vi "2P_AdapUprite_Linlin.vi"() -> ()   [LabVIEW 2015] (continued)
                        n4091 = control-ref of="Digital Lines Plot"() -> (w894:refnum<vi>)
                        n4092 = local write "Digital Used Lines"(w892) -> ()
                        n4093 = local write "Digital Used Names"(w893) -> ()
                        n4094 = call "prepAOWaveplot.vi"("WaveformGraph in"=w896, "Analog Used Names"=w895) -> ()  [unwired: 1 in]
                        n4095 = call "prepDOWaveplot.vi"("DigitalGraph in"=w894, "used DO names"=w893) -> ()  [unwired: 1 in]
                      }
                    }
                  }
                  frame #4 {
                    n4096 = local read "remDO"() -> (w899:bool)
                    n4097 = case shown="True" w899 {
                      tunnel: w898 -> [_ w900]
                      frame False {
                      }
                      frame True {
                        n4098 = call "waveformparamsv2.vi"("command"="rem DO", "index"=w900) -> ()  [unwired: 3 in, 3 out]
                      }
                    }
                  }
                  frame #5 {
                    n4099 = local read "Meastab"() -> (w905:enum32{"X-Y Image", "Linescan", "Timetrace"})
                    n4100 = property on="refwf" class="Ring (strict)"() -> ("RingText.Text"=w912:string)  [unwired: 2 in, 2 out]
                    n4101 = call "waveformsDObuffer.vi"("command"="get") -> ("DO wf out"=w911:digitalwaveform[])  [unwired: 1 in]
                    n4102 = case shown="\"Timetrace\"" w905 {
                      tunnel: [w921 w922] -> w904
                      frame "X-Y Image", Default {
                        n4103 = local read "Sampling rate"() -> (w921:dbl)
                      }
                      frame "Timetrace" {
                        n4104 = local read "srateAODOtt"() -> (w922:dbl)
                      }
                    }
                    n4105 = call "waveformsAObuffer.vi"("command"="get") -> ("AO wf out"=w920:waveform(dbl)[])  [unwired: 1 in]
                    n4106 = Delete From Array(array=w911, length=1, index=w909) -> (array with subset deleted=w908:digitalwaveform[])  [unwired: 1 out]
                    n4107 = call "correctwaveformsizetemp.vi"("new sampling frequency (Hz)"=w904, "start"=FALSE, "reference waveforms to"=w912, "Analog waveforms in"=w920, "stop"=FALSE, "Digital waveforms in"=w908) -> ("analog wf out"=w915:waveform(dbl)[], "Digital wf out"=w913:digitalwaveform[], "measpoints"=w906:i32)
                    n4108 = local read "wavdet"() -> (w907:bool)
                    n4109 = call "waveformsAObuffer.vi"("AO wf in"=w915, "command"="set") -> ()  [unwired: 1 out]
                    n4110 = call "waveformsDObuffer.vi"("DO wf in"=w913, "command"="set") -> ()  [unwired: 1 out]
                    n4111 = local write "Analog Lines Plot"(w915) -> ()
                    n4112 = local write "Digital Lines Plot"(w913) -> ()
                    n4113 = call "GetNumCamFramesv2.vi"("Digital Waveform Graph"=w913) -> ("Numeric"=w914:i32)  [unwired: 10 in]
                    n4114 = case shown="True" w907 {
                      tunnel: w906 -> [_ w923]
                      frame False {
                      }
                      frame True {
                        n4115 = local write "# of frames"(w923) -> ()
                      }
                    }
                    n4116 = local write "Total Camera Frames"(w914) -> ()
                  }
                  frame #6 {
                    w924 = FALSE ("addAO")
                    n4117 = local read "finite samples"() -> (w925:bool)
                    n4118 = local read "continuous"() -> (w926:bool)
                    n4119 = local read "wavdet"() -> (w927:bool)
                    n4120 = local write "remDO"(w924) -> ()
                    n4121 = call "2pparameters.vi"("command"="get") -> ("params out"=w930:T12)  [unwired: 1 in]
                    n4122 = Bundle By Name(cluster=w930, "finite"=w925, "cont"=w926, "wavdet"=w927) -> (w928:T12)
                    n4123 = property on="Rem DO wave" class="Bool (strict)"("Val(Sgnl)"=w924) -> ()  [unwired: 2 in, 2 out]
                    n4124 = call "2pparameters.vi"("Params in"=w928, "command"="set") -> ()  [unwired: 1 out]
                  }
                }
              }
            }
          }
          event "load changed DO wave": Value Change {
            n4125 = event-data() -> ("NewVal"=w932:bool)  [unwired: 1 in, 5 out]
            n4126 = case shown="True" w932 {
              frame False {
              }
              frame True {
                n4127 = stacked-sequence {
                  seq-local: [_ _ w1040 _ _] -> [_ _ _ w1057 _]
                  seq-local: [_ _ w1039 _ _] -> [_ _ _ w1056 _]
                  frame #0 {
                    n4128 = local read "Measurement"() -> (w934:T4)
                    n4129 = local write "changeDO"(TRUE ("addAO")) -> ()
                    n4130 = case shown="\"X-Y-t movie\", Default" w934 {
                      frame "X-Y-t movie", Default {
                        n4131 = local read "avpp"() -> (w955:i32)
                        n4132 = local read "Angle ref"() -> (w954:dbl)
                        n4133 = local read "ROI Type"() -> (w953:u16)
                        n4134 = local read "xpixels ref"() -> (w950:i32)
                        n4135 = local read "Vx-min ref"() -> (w949:dbl)
                        n4136 = local read "Vx-max ref"() -> (w948:dbl)
                        n4137 = local read "ypixels ref"() -> (w946:i32)
                        n4138 = local read "Vy-min ref"() -> (w947:dbl)
                        n4139 = local read "Vy-max ref"() -> (w943:dbl)
                        n4140 = local read "Sampling rate"() -> (w937:dbl)
                        n4141 = local read "finite samples"() -> (w938:bool)
                        n4142 = local read "continuous"() -> (w941:bool)
                        n4143 = local read "wavdet"() -> (w942:bool)
                        n4144 = local read "# of frames"() -> (w940:i32)
                        n4145 = local read "maxbufferAI"() -> (w939:i32)
                        n4146 = local read "Override AI buffer"() -> (w935:bool)
                        n4147 = call "2pparameters.vi"("command"="get") -> ("params out"=w952:T12)  [unwired: 1 in]
                        n4148 = Bundle By Name(cluster=w952, "type"="X-Y-t movie", "avpp"=w955, "Angle Img"=w954, "Xpixels Img"=w950, "Vx-min Img"=w949, "VX-max Img"=w948, "Ypixels Img"=w946, "Vy-min Img"=w947, "Vy-max Img"=w943, "srate"=w937, "srate Img"=w937, "finite"=w938, "cont"=w941, "wavdet"=w942, "measpoints"=w940, "maxbufferAI"=w939, "Drawing Mode"=w953, "Vz-reset"=0.0, "AIoverride"=w935) -> (w944:T12)
                        n4149 = call "2pparameters.vi"("Params in"=w944, "command"="set") -> ()  [unwired: 1 out]
                      }
                      frame "X-Y-Z stack" {
                        n4150 = call "2pparameters.vi"("command"="get") -> ("params out"=w959:T12)  [unwired: 1 in]
                        n4151 = Bundle By Name(cluster=w959, "type"="X-Y-Z stack") -> (w957:T12)
                        n4152 = call "2pparameters.vi"("Params in"=w957, "command"="set") -> ()  [unwired: 1 out]
                      }
                      frame "Lifetime (scan)" {
                        n4153 = call "2pparameters.vi"("command"="get") -> ("params out"=w964:T12)  [unwired: 1 in]
                        n4154 = Bundle By Name(cluster=w964, "type"="Lifetime (scan)") -> (w962:T12)
                        n4155 = call "2pparameters.vi"("Params in"=w962, "command"="set") -> ()  [unwired: 1 out]
                      }
                      frame "Lifetime (contour)" {
                        n4156 = local read "Vy-min draw"() -> (w974:dbl)
                        n4157 = local read "Vy-max draw"() -> (w973:dbl)
                        n4158 = local read "Vx-min draw"() -> (w976:dbl)
                        n4159 = local read "Vx-max draw"() -> (w975:dbl)
                        n4160 = local read "xpixels ref"() -> (w972:i32)
                        n4161 = local read "ypixels ref"() -> (w971:i32)
                        n4162 = local read "ROI Type"() -> (w970:u16)
                        n4163 = local read "srateAODOtt"() -> (w981:dbl)
                        n4164 = local read "# of frames"() -> (w986:i32)
                        n4165 = local read "refreshtime"() -> (w978:dbl)
                        n4166 = local read "Pel"() -> (w969:dbl)
                        n4167 = local read "bin"() -> (w984:dbl)
                        n4168 = local read "Override AI buffer"() -> (w967:bool)
                        n4169 = local read "finite samples"() -> (w993:bool)
                        n4170 = local read "srateAODOtt"() -> (w980:dbl)
                        n4171 = local read "srateAODOtt"() -> (w987:dbl)
                        n4172 = local read "continuous"() -> (w992:bool)
                        n4173 = local read "Angle ref"() -> (w977:dbl)
                        n4174 = local read "wavdet"() -> (w994:bool)
                        n4175 = local read "Vx-ref"() -> (w989:dbl)
                        n4176 = local read "Vy-ref"() -> (w991:dbl)
                        n4177 = local read "avpp"() -> (w990:i32)
                        n4178 = call "tt_timeandsamples.vi"("bin"=w984, "refreshtime"=w978, "srateAODOtt"=w981, "tot#ofsamples"=w986) -> ("refreshrate"=w982:dbl, "refreshbuffer"=w983:i32, "timetracecycles"=w988:i32)  [unwired: 5 in]
                        n4179 = local read "bin"() -> (w985:dbl)
                        n4180 = call "2pparameters.vi"("command"="get") -> ("params out"=w997:T12)  [unwired: 1 in]
                        n4181 = Bundle By Name(cluster=w997, "Drawing Mode"=w970, "measpoints"=w986, "tt_cycles"=w988, "refreshbuffer"=w983, "refreshrate"=w982, "Vx-ref"=w989, "Vy-ref"=w991, "srate"=w980, "finite"=w993, "cont"=w992, "wavdet"=w994, "avpp"=w990, "srateAODO"=w987, "bufferAI"=w983, "bin"=w985, "Angle Img"=w977, "Vxminref"=w976, "Vxmaxref"=w975, "Vyminref"=w974, "Vymaxref"=w973, "Xpixels Img"=w972, "Ypixels Img"=w971, "Pel"=w969, "Vz-reset"=0.0, "AIoverride"=w967, "type"="Lifetime (contour)") -> (w995:T12)
                        n4182 = Reciprocal(x=w982) -> (1/x=w979:dbl)
                        n4183 = local write "refreshtime"(w979) -> ()
                        n4184 = call "2pparameters.vi"("Params in"=w995, "command"="set") -> ()  [unwired: 1 out]
                      }
                      frame "X-Y-Z-t movie" {
                      }
                      frame "linescan" {
                      }
                      frame "Timetrace" {
                        n4185 = local read "Vy-min draw"() -> (w1007:dbl)
                        n4186 = local read "Vy-max draw"() -> (w1006:dbl)
                        n4187 = local read "Vx-min draw"() -> (w1009:dbl)
                        n4188 = local read "Vx-max draw"() -> (w1008:dbl)
                        n4189 = local read "xpixels ref"() -> (w1005:i32)
                        n4190 = local read "ypixels ref"() -> (w1004:i32)
                        n4191 = local read "ROI Type"() -> (w1003:u16)
                        n4192 = local read "srateAODOtt"() -> (w1014:dbl)
                        n4193 = local read "# of frames"() -> (w1019:i32)
                        n4194 = local read "refreshtime"() -> (w1011:dbl)
                        n4195 = local read "Pel"() -> (w1002:dbl)
                        n4196 = local read "bin"() -> (w1017:dbl)
                        n4197 = local read "Override AI buffer"() -> (w1000:bool)
                        n4198 = local read "finite samples"() -> (w1026:bool)
                        n4199 = local read "srateAODOtt"() -> (w1013:dbl)
                        n4200 = local read "srateAODOtt"() -> (w1020:dbl)
                        n4201 = local read "continuous"() -> (w1025:bool)
                        n4202 = local read "Angle ref"() -> (w1010:dbl)
                        n4203 = local read "wavdet"() -> (w1027:bool)
                        n4204 = local read "Vx-ref"() -> (w1022:dbl)
                        n4205 = local read "Vy-ref"() -> (w1024:dbl)
                        n4206 = local read "avpp"() -> (w1023:i32)
                        n4207 = call "tt_timeandsamples.vi"("bin"=w1017, "refreshtime"=w1011, "srateAODOtt"=w1014, "tot#ofsamples"=w1019) -> ("refreshrate"=w1015:dbl, "refreshbuffer"=w1016:i32, "timetracecycles"=w1021:i32)  [unwired: 5 in]
                        n4208 = local read "bin"() -> (w1018:dbl)
                        n4209 = call "2pparameters.vi"("command"="get") -> ("params out"=w1030:T12)  [unwired: 1 in]
                        n4210 = Bundle By Name(cluster=w1030, "Drawing Mode"=w1003, "measpoints"=w1019, "tt_cycles"=w1021, "refreshbuffer"=w1016, "refreshrate"=w1015, "Vx-ref"=w1022, "Vy-ref"=w1024, "srate"=w1013, "finite"=w1026, "cont"=w1025, "wavdet"=w1027, "avpp"=w1023, "srateAODO"=w1020, "bufferAI"=w1016, "bin"=w1018, "Angle Img"=w1010, "Vxminref"=w1009, "Vxmaxref"=w1008, "Vyminref"=w1007, "Vymaxref"=w1006, "Xpixels Img"=w1005, "Ypixels Img"=w1004, "Pel"=w1002, "Vz-reset"=0.0, "AIoverride"=w1000, "type"="Timetrace") -> (w1028:T12)
                        n4211 = Reciprocal(x=w1015) -> (1/x=w1012:dbl)
                        n4212 = local write "refreshtime"(w1012) -> ()
                        n4213 = call "2pparameters.vi"("Params in"=w1028, "command"="set") -> ()  [unwired: 1 out]
                      }
                      frame "Lifetime (point)" {
                      }
                    }
                  }
                  frame #1 {
                    w1033 = FALSE ("wavdet")
                    n4214 = call "2pparameters.vi"("command"="get") -> ("params out"=w1037:T12)  [unwired: 1 in]
                    n4215 = Bundle By Name(cluster=w1037, "finite"=w1033, "cont"=w1033, "wavdet"=TRUE) -> (w1034:T12)
                    n4216 = call "2pparameters.vi"("Params in"=w1034, "command"="set") -> ()  [unwired: 1 out]
                  }
                  frame #2 {
                    n4217 = local read "DO channels"() -> (w1042:u16)
                    n4218 = call "2pparameters.vi"("command"="get") -> ("params out"=w1044:T12)  [unwired: 1 in]
                    n4219 = Unbundle By Name(w1044) -> ("aDO"=w1043:u32[])
                    n4220 = Search 1D Array(1D array=w1043, element=w1042) -> (index of element=w1040:i32)  [unwired: 1 in]
                    n4221 = Greater?(x=w1040, y=-1) -> (0:w1039:bool)
                    n4222 = case shown="True" w1039 {
                      tunnel: w1040 -> [_ w1053]
                      frame False {
                      }
                      frame True {
                        n4223 = local read "Meastab"() -> (w1047:enum32{"X-Y Image", "Linescan", "Timetrace"})
                        n4224 = local read "Digital padding value"() -> (w1048:dbl)
                        n4225 = local read "Digital time offset (s)"() -> (w1049:dbl)
                        n4226 = case shown="\"Timetrace\"" w1047 {
                          tunnel: [w1054 w1055] -> w1046
                          frame "X-Y Image", Default {
                            n4227 = local read "Sampling rate"() -> (w1054:dbl)
                          }
                          frame "Timetrace" {
                            n4228 = local read "srateAODOtt"() -> (w1055:dbl)
                          }
                        }
                        n4229 = local read "Digital Freq (Hz)"() -> (w1051:dbl)
                        n4230 = local read "Digital phase (s)"() -> (w1050:dbl)
                        n4231 = local read "Digital DC (%)"() -> (w1052:dbl)
                        n4232 = call "replace DO wf param.vi"("Digital Freq (Hz)"=w1051, "Digital DC (%)"=w1052, "Digital phase"=w1050, "Sampling frequency (Hz)"=w1046, "Digital time offset (s)"=w1049, "index of DO wave"=w1053, "padding value"=w1048) -> ()  [unwired: 4 in]
                      }
                    }
                  }
                  frame #3 {
                    n4233 = case shown="True" w1056 {
                      tunnel: w1057 -> [_ w1064]
                      frame False {
                      }
                      frame True {
                        n4234 = local read "Meastab"() -> (w1061:enum32{"X-Y Image", "Linescan", "Timetrace"})
                        n4235 = call "waveformparamsv2.vi"("command"="get") -> ("Params out"=w1080:T17)  [unwired: 4 in, 2 out]
                        n4236 = Unbundle By Name(w1080) -> ("DO parameters"=w1079:T20)
                        n4237 = property on="refwf" class="Ring (strict)"() -> ("RingText.Text"=w1086:string)  [unwired: 2 in, 2 out]
                        n4238 = case shown="\"Timetrace\"" w1061 {
                          tunnel: [w1087 w1088] -> w1060
                          frame "X-Y Image", Default {
                            n4239 = local read "Sampling rate"() -> (w1087:dbl)
                          }
                          frame "Timetrace" {
                            n4240 = local read "srateAODOtt"() -> (w1088:dbl)
                          }
                        }
                        n4241 = call "waveformsAObuffer.vi"("command"="get") -> ("AO wf out"=w1084:waveform(dbl)[])  [unwired: 1 in]
                        n4242 = call "waveformsDObuffer.vi"("command"="get") -> ("DO wf out"=w1082:digitalwaveform[])  [unwired: 1 in]
                        n4243 = call "referfencesize.vi"("Digital waveforms in"=w1082, "Analog waveforms in"=w1084, "reference waveforms to"=w1086) -> ("number of samples"=w1077:i32)  [unwired: 2 in]
                        n4244 = Index Array(array=w1079, index=w1064) -> (element=w1078:T21)
                        n4245 = call "waveformsDObuffer.vi"("command"="get") -> ("DO wf out"=w1074:digitalwaveform[])  [unwired: 1 in]
                        n4246 = call "simple digital from wf params.vi"("waveform params"=w1078, "number of samples"=w1077) -> ("digital waveform"=w1076:digitalwaveform)
                        n4247 = property on="refwf" class="Ring (strict)"() -> ("RingText.Text"=w1066:string)  [unwired: 2 in, 2 out]
                        n4248 = Replace Array Subset(array=w1074, new element=w1076, index=w1064) -> (w1065:digitalwaveform[])
                        n4249 = call "waveformsAObuffer.vi"("command"="get") -> ("AO wf out"=w1073:waveform(dbl)[])  [unwired: 1 in]
                        n4250 = local read "wavdet"() -> (w1063:bool)
                        n4251 = call "correctwaveformsizetemp.vi"("new sampling frequency (Hz)"=w1060, "start"=FALSE, "reference waveforms to"=w1066, "Analog waveforms in"=w1073, "stop"=FALSE, "Digital waveforms in"=w1065) -> ("analog wf out"=w1069:waveform(dbl)[], "Digital wf out"=w1067:digitalwaveform[], "measpoints"=w1062:i32)
                        n4252 = local write "Analog Lines Plot"(w1069) -> ()
                        n4253 = call "GetNumCamFramesv2.vi"("Digital Waveform Graph"=w1067) -> ("Numeric"=w1068:i32)  [unwired: 10 in]
                        n4254 = local write "Digital Lines Plot"(w1067) -> ()
                        n4255 = case shown="True" w1063 {
                          tunnel: w1062 -> [_ w1089]
                          frame False {
                          }
                          frame True {
                            n4256 = local write "# of frames"(w1089) -> ()
                          }
                        }
                        n4257 = call "waveformsAObuffer.vi"("AO wf in"=w1069, "command"="set") -> ()  [unwired: 1 out]
                        n4258 = call "waveformsDObuffer.vi"("DO wf in"=w1067, "command"="set") -> ()  [unwired: 1 out]
                        n4259 = local write "Total Camera Frames"(w1068) -> ()
                      }
                    }
                  }
                  frame #4 {
                    w1091 = FALSE ("addAO")
                    n4260 = local read "finite samples"() -> (w1092:bool)
                    n4261 = local read "continuous"() -> (w1093:bool)
                    n4262 = local read "wavdet"() -> (w1094:bool)
                    n4263 = local write "changeDO"(w1091) -> ()
                    n4264 = property on="load changed DO wave" class="Bool (strict)"("Val(Sgnl)"=w1091) -> ()  [unwired: 2 in, 2 out]
                    n4265 = call "2pparameters.vi"("command"="get") -> ("params out"=w1097:T12)  [unwired: 1 in]
                    n4266 = Bundle By Name(cluster=w1097, "finite"=w1092, "cont"=w1093, "wavdet"=w1094) -> (w1095:T12)
                    n4267 = local write "not loadedDO"(FALSE ("not loadedDO")) -> ()
                    n4268 = call "2pparameters.vi"("Params in"=w1095, "command"="set") -> ()  [unwired: 1 out]
                  }
                }
              }
            }
          }
          event "refwf": Value Change {
            n4269 = event-data() -> ()  [unwired: 1 in, 6 out]
            n4270 = stacked-sequence {
              frame #0 {
                n4271 = local read "Measurement"() -> (w1099:T4)
                n4272 = case shown="\"Timetrace\"" w1099 {
                  frame "X-Y-t movie", Default {
                    n4273 = local read "avpp"() -> (w1120:i32)
                    n4274 = local read "Angle ref"() -> (w1119:dbl)
                    n4275 = local read "ROI Type"() -> (w1118:u16)
                    n4276 = local read "xpixels ref"() -> (w1115:i32)
                    n4277 = local read "Vx-min ref"() -> (w1114:dbl)
                    n4278 = local read "Vx-max ref"() -> (w1113:dbl)
                    n4279 = local read "ypixels ref"() -> (w1111:i32)
                    n4280 = local read "Vy-min ref"() -> (w1112:dbl)
                    n4281 = local read "Vy-max ref"() -> (w1108:dbl)
                    n4282 = local read "Sampling rate"() -> (w1102:dbl)
                    n4283 = local read "finite samples"() -> (w1103:bool)
                    n4284 = local read "continuous"() -> (w1106:bool)
                    n4285 = local read "wavdet"() -> (w1107:bool)
                    n4286 = local read "# of frames"() -> (w1105:i32)
                    n4287 = local read "maxbufferAI"() -> (w1104:i32)
                    n4288 = local read "Override AI buffer"() -> (w1100:bool)
                    n4289 = call "2pparameters.vi"("command"="get") -> ("params out"=w1117:T12)  [unwired: 1 in]
                    n4290 = Bundle By Name(cluster=w1117, "type"="X-Y-t movie", "avpp"=w1120, "Angle Img"=w1119, "Xpixels Img"=w1115, "Vx-min Img"=w1114, "VX-max Img"=w1113, "Ypixels Img"=w1111, "Vy-min Img"=w1112, "Vy-max Img"=w1108, "srate"=w1102, "srate Img"=w1102, "finite"=w1103, "cont"=w1106, "wavdet"=w1107, "measpoints"=w1105, "maxbufferAI"=w1104, "Drawing Mode"=w1118, "Vz-reset"=0.0, "AIoverride"=w1100) -> (w1109:T12)
                    n4291 = call "2pparameters.vi"("Params in"=w1109, "command"="set") -> ()  [unwired: 1 out]
                  }
                  frame "X-Y-Z stack" {
                    n4292 = call "2pparameters.vi"("command"="get") -> ("params out"=w1124:T12)  [unwired: 1 in]
                    n4293 = Bundle By Name(cluster=w1124, "type"="X-Y-Z stack") -> (w1122:T12)
                    n4294 = call "2pparameters.vi"("Params in"=w1122, "command"="set") -> ()  [unwired: 1 out]
                  }
                  frame "Lifetime (scan)" {
                    n4295 = call "2pparameters.vi"("command"="get") -> ("params out"=w1129:T12)  [unwired: 1 in]
                    n4296 = Bundle By Name(cluster=w1129, "type"="Lifetime (scan)") -> (w1127:T12)
                    n4297 = call "2pparameters.vi"("Params in"=w1127, "command"="set") -> ()  [unwired: 1 out]
                  }
                  frame "Lifetime (contour)" {
                    n4298 = local read "Vy-min draw"() -> (w1139:dbl)
                    n4299 = local read "Vy-max draw"() -> (w1138:dbl)
                    n4300 = local read "Vx-min draw"() -> (w1141:dbl)
                    n4301 = local read "Vx-max draw"() -> (w1140:dbl)
                    n4302 = local read "xpixels ref"() -> (w1137:i32)
                    n4303 = local read "ypixels ref"() -> (w1136:i32)
                    n4304 = local read "ROI Type"() -> (w1135:u16)
                    n4305 = local read "srateAODOtt"() -> (w1146:dbl)
                    n4306 = local read "# of frames"() -> (w1151:i32)
                    n4307 = local read "refreshtime"() -> (w1143:dbl)
                    n4308 = local read "Pel"() -> (w1134:dbl)
                    n4309 = local read "bin"() -> (w1149:dbl)
                    n4310 = local read "Override AI buffer"() -> (w1132:bool)
                    n4311 = local read "finite samples"() -> (w1158:bool)
                    n4312 = local read "srateAODOtt"() -> (w1145:dbl)
                    n4313 = local read "srateAODOtt"() -> (w1152:dbl)
                    n4314 = local read "continuous"() -> (w1157:bool)
                    n4315 = local read "Angle ref"() -> (w1142:dbl)
                    n4316 = local read "wavdet"() -> (w1159:bool)
                    n4317 = local read "Vx-ref"() -> (w1154:dbl)
                    n4318 = local read "Vy-ref"() -> (w1156:dbl)
                    n4319 = local read "avpp"() -> (w1155:i32)
                    n4320 = call "tt_timeandsamples.vi"("bin"=w1149, "refreshtime"=w1143, "srateAODOtt"=w1146, "tot#ofsamples"=w1151) -> ("refreshrate"=w1147:dbl, "refreshbuffer"=w1148:i32, "timetracecycles"=w1153:i32)  [unwired: 5 in]
                    n4321 = local read "bin"() -> (w1150:dbl)
                    n4322 = call "2pparameters.vi"("command"="get") -> ("params out"=w1162:T12)  [unwired: 1 in]
                    n4323 = Bundle By Name(cluster=w1162, "Drawing Mode"=w1135, "measpoints"=w1151, "tt_cycles"=w1153, "refreshbuffer"=w1148, "refreshrate"=w1147, "Vx-ref"=w1154, "Vy-ref"=w1156, "srate"=w1145, "finite"=w1158, "cont"=w1157, "wavdet"=w1159, "avpp"=w1155, "srateAODO"=w1152, "bufferAI"=w1148, "bin"=w1150, "Angle Img"=w1142, "Vxminref"=w1141, "Vxmaxref"=w1140, "Vyminref"=w1139, "Vymaxref"=w1138, "Xpixels Img"=w1137, "Ypixels Img"=w1136, "Pel"=w1134, "Vz-reset"=0.0, "AIoverride"=w1132, "type"="Lifetime (contour)") -> (w1160:T12)
                    n4324 = Reciprocal(x=w1147) -> (1/x=w1144:dbl)
                    n4325 = local write "refreshtime"(w1144) -> ()
                    n4326 = call "2pparameters.vi"("Params in"=w1160, "command"="set") -> ()  [unwired: 1 out]
                  }
                  frame "X-Y-Z-t movie" {
                  }
                  frame "linescan" {
                  }
                  frame "Timetrace" {
                    n4327 = local read "Vy-min draw"() -> (w1172:dbl)
                    n4328 = local read "Vy-max draw"() -> (w1171:dbl)
                    n4329 = local read "Vx-min draw"() -> (w1174:dbl)
                    n4330 = local read "Vx-max draw"() -> (w1173:dbl)
                    n4331 = local read "xpixels ref"() -> (w1170:i32)
                    n4332 = local read "ypixels ref"() -> (w1169:i32)
                    n4333 = local read "ROI Type"() -> (w1168:u16)
                    n4334 = local read "srateAODOtt"() -> (w1179:dbl)
                    n4335 = local read "# of frames"() -> (w1184:i32)
                    n4336 = local read "refreshtime"() -> (w1176:dbl)
                    n4337 = local read "Pel"() -> (w1167:dbl)
                    n4338 = local read "bin"() -> (w1182:dbl)
                    n4339 = local read "Override AI buffer"() -> (w1165:bool)
                    n4340 = local read "finite samples"() -> (w1191:bool)
                    n4341 = local read "srateAODOtt"() -> (w1178:dbl)
                    n4342 = local read "srateAODOtt"() -> (w1185:dbl)
                    n4343 = local read "continuous"() -> (w1190:bool)
                    n4344 = local read "Angle ref"() -> (w1175:dbl)
                    n4345 = local read "wavdet"() -> (w1192:bool)
                    n4346 = local read "Vx-ref"() -> (w1187:dbl)
                    n4347 = local read "Vy-ref"() -> (w1189:dbl)
                    n4348 = local read "avpp"() -> (w1188:i32)
                    n4349 = call "tt_timeandsamples.vi"("bin"=w1182, "refreshtime"=w1176, "srateAODOtt"=w1179, "tot#ofsamples"=w1184) -> ("refreshrate"=w1180:dbl, "refreshbuffer"=w1181:i32, "timetracecycles"=w1186:i32)  [unwired: 5 in]
                    n4350 = local read "bin"() -> (w1183:dbl)
                    n4351 = call "2pparameters.vi"("command"="get") -> ("params out"=w1195:T12)  [unwired: 1 in]
                    n4352 = Bundle By Name(cluster=w1195, "Drawing Mode"=w1168, "measpoints"=w1184, "tt_cycles"=w1186, "refreshbuffer"=w1181, "refreshrate"=w1180, "Vx-ref"=w1187, "Vy-ref"=w1189, "srate"=w1178, "finite"=w1191, "cont"=w1190, "wavdet"=w1192, "avpp"=w1188, "srateAODO"=w1185, "bufferAI"=w1181, "bin"=w1183, "Angle Img"=w1175, "Vxminref"=w1174, "Vxmaxref"=w1173, "Vyminref"=w1172, "Vymaxref"=w1171, "Xpixels Img"=w1170, "Ypixels Img"=w1169, "Pel"=w1167, "Vz-reset"=0.0, "AIoverride"=w1165, "type"="Timetrace") -> (w1193:T12)
                    n4353 = Reciprocal(x=w1180) -> (1/x=w1177:dbl)
                    n4354 = local write "refreshtime"(w1177) -> ()
                    n4355 = call "2pparameters.vi"("Params in"=w1193, "command"="set") -> ()  [unwired: 1 out]
                  }
                  frame "Lifetime (point)" {
                  }
                }
              }
              frame #1 {
                w1198 = FALSE ("wavdet")
                n4356 = call "2pparameters.vi"("command"="get") -> ("params out"=w1202:T12)  [unwired: 1 in]
                n4357 = Bundle By Name(cluster=w1202, "finite"=w1198, "cont"=w1198, "wavdet"=TRUE) -> (w1199:T12)
                n4358 = call "2pparameters.vi"("Params in"=w1199, "command"="set") -> ()  [unwired: 1 out]
              }
              frame #2 {
                n4359 = local read "Meastab"() -> (w1207:enum32{"X-Y Image", "Linescan", "Timetrace"})
                n4360 = property on="refwf" class="Ring (strict)"() -> ("RingText.Text"=w1210:string)  [unwired: 2 in, 2 out]
                n4361 = case shown="\"Timetrace\"" w1207 {
                  tunnel: [w1220 w1221] -> w1206
                  frame "X-Y Image", Default {
                    n4362 = local read "Sampling rate"() -> (w1220:dbl)
                  }
                  frame "Timetrace" {
                    n4363 = local read "srateAODOtt"() -> (w1221:dbl)
                  }
                }
                n4364 = call "waveformsAObuffer.vi"("command"="get") -> ("AO wf out"=w1219:waveform(dbl)[])  [unwired: 1 in]
                n4365 = local read "wavdet"() -> (w1209:bool)
                n4366 = call "waveformsDObuffer.vi"("command"="get") -> ("DO wf out"=w1215:digitalwaveform[])  [unwired: 1 in]
                n4367 = call "correctwaveformsizetemp.vi"("new sampling frequency (Hz)"=w1206, "start"=FALSE, "reference waveforms to"=w1210, "Analog waveforms in"=w1219, "stop"=FALSE, "Digital waveforms in"=w1215) -> ("analog wf out"=w1213:waveform(dbl)[], "Digital wf out"=w1211:digitalwaveform[], "measpoints"=w1208:i32)
                n4368 = local write "Analog Lines Plot"(w1213) -> ()
                n4369 = call "GetNumCamFramesv2.vi"("Digital Waveform Graph"=w1211) -> ("Numeric"=w1212:i32)  [unwired: 10 in]
                n4370 = local write "Digital Lines Plot"(w1211) -> ()
                n4371 = call "waveformsDObuffer.vi"("DO wf in"=w1211, "command"="set") -> ()  [unwired: 1 out]
                n4372 = call "waveformsAObuffer.vi"("AO wf in"=w1213, "command"="set") -> ()  [unwired: 1 out]
                n4373 = local write "Total Camera Frames"(w1212) -> ()
                n4374 = case shown="True" w1209 {
                  tunnel: w1208 -> [_ w1222]
                  frame False {
                  }
                  frame True {
                    n4375 = local write "# of frames"(w1222) -> ()
                  }
                }
              }
              frame #3 {
                n4376 = local read "finite samples"() -> (w1223:bool)
                n4377 = local read "continuous"() -> (w1224:bool)
                n4378 = local read "wavdet"() -> (w1225:bool)
                n4379 = call "2pparameters.vi"("command"="get") -> ("params out"=w1228:T12)  [unwired: 1 in]
                n4380 = Bundle By Name(cluster=w1228, "finite"=w1223, "cont"=w1224, "wavdet"=w1225) -> (w1226:T12)
                n4381 = call "2pparameters.vi"("Params in"=w1226, "command"="set") -> ()  [unwired: 1 out]
              }
            }
          }
          event "load changed AOsq": Value Change {
            n4382 = event-data() -> ("NewVal"=w1230:bool)  [unwired: 1 in, 5 out]
            n4383 = case shown="True" w1230 {
              frame False {
              }
              frame True {
                n4384 = stacked-sequence {
                  seq-local: [_ _ _ w1372 _ _] -> [_ _ _ _ w1397 _]
                  seq-local: [_ _ _ w1371 _ _] -> [_ _ _ _ w1396 _]
                  seq-local: [_ _ w1338 _ _ _] -> [_ _ _ w1370 w1395 w1426]
                  frame #0 {
                    n4385 = local read "Measurement"() -> (w1232:T4)
                    n4386 = local write "changeAOsq"(TRUE ("addAO")) -> ()
                    n4387 = case shown="\"X-Y-t movie\", Default" w1232 {
                      frame "X-Y-t movie", Default {
                        n4388 = local read "avpp"() -> (w1253:i32)
                        n4389 = local read "Angle ref"() -> (w1252:dbl)
                        n4390 = local read "ROI Type"() -> (w1251:u16)
                        n4391 = local read "xpixels ref"() -> (w1248:i32)
                        n4392 = local read "Vx-min ref"() -> (w1247:dbl)
                        n4393 = local read "Vx-max ref"() -> (w1246:dbl)
                        n4394 = local read "ypixels ref"() -> (w1244:i32)
                        n4395 = local read "Vy-min ref"() -> (w1245:dbl)
                        n4396 = local read "Vy-max ref"() -> (w1241:dbl)
                        n4397 = local read "Sampling rate"() -> (w1235:dbl)
                        n4398 = local read "finite samples"() -> (w1236:bool)
                        n4399 = local read "continuous"() -> (w1239:bool)
                        n4400 = local read "wavdet"() -> (w1240:bool)
                        n4401 = local read "# of frames"() -> (w1238:i32)
                        n4402 = local read "maxbufferAI"() -> (w1237:i32)
                        n4403 = local read "Override AI buffer"() -> (w1233:bool)
                        n4404 = call "2pparameters.vi"("command"="get") -> ("params out"=w1250:T12)  [unwired: 1 in]
                        n4405 = Bundle By Name(cluster=w1250, "type"="X-Y-t movie", "avpp"=w1253, "Angle Img"=w1252, "Xpixels Img"=w1248, "Vx-min Img"=w1247, "VX-max Img"=w1246, "Ypixels Img"=w1244, "Vy-min Img"=w1245, "Vy-max Img"=w1241, "srate"=w1235, "srate Img"=w1235, "finite"=w1236, "cont"=w1239, "wavdet"=w1240, "measpoints"=w1238, "maxbufferAI"=w1237, "Drawing Mode"=w1251, "Vz-reset"=0.0, "AIoverride"=w1233) -> (w1242:T12)
                        n4406 = call "2pparameters.vi"("Params in"=w1242, "command"="set") -> ()  [unwired: 1 out]
                      }
                      frame "X-Y-Z stack" {
                        n4407 = call "2pparameters.vi"("command"="get") -> ("params out"=w1257:T12)  [unwired: 1 in]
                        n4408 = Bundle By Name(cluster=w1257, "type"="X-Y-Z stack") -> (w1255:T12)
                        n4409 = call "2pparameters.vi"("Params in"=w1255, "command"="set") -> ()  [unwired: 1 out]
                      }
                      frame "Lifetime (scan)" {
                        n4410 = call "2pparameters.vi"("command"="get") -> ("params out"=w1262:T12)  [unwired: 1 in]
                        n4411 = Bundle By Name(cluster=w1262, "type"="Lifetime (scan)") -> (w1260:T12)
                        n4412 = call "2pparameters.vi"("Params in"=w1260, "command"="set") -> ()  [unwired: 1 out]
                      }
                      frame "Lifetime (contour)" {
                        n4413 = local read "Vy-min draw"() -> (w1272:dbl)
                        n4414 = local read "Vy-max draw"() -> (w1271:dbl)
                        n4415 = local read "Vx-min draw"() -> (w1274:dbl)
                        n4416 = local read "Vx-max draw"() -> (w1273:dbl)
                        n4417 = local read "xpixels ref"() -> (w1270:i32)
                        n4418 = local read "ypixels ref"() -> (w1269:i32)
                        n4419 = local read "ROI Type"() -> (w1268:u16)
                        n4420 = local read "srateAODOtt"() -> (w1279:dbl)
                        n4421 = local read "# of frames"() -> (w1284:i32)
                        n4422 = local read "refreshtime"() -> (w1276:dbl)
                        n4423 = local read "Pel"() -> (w1267:dbl)
                        n4424 = local read "bin"() -> (w1282:dbl)
                        n4425 = local read "Override AI buffer"() -> (w1265:bool)
                        n4426 = local read "finite samples"() -> (w1291:bool)
                        n4427 = local read "srateAODOtt"() -> (w1278:dbl)
                        n4428 = local read "srateAODOtt"() -> (w1285:dbl)
                        n4429 = local read "continuous"() -> (w1290:bool)
                        n4430 = local read "Angle ref"() -> (w1275:dbl)
                        n4431 = local read "wavdet"() -> (w1292:bool)
                        n4432 = local read "Vx-ref"() -> (w1287:dbl)
                        n4433 = local read "Vy-ref"() -> (w1289:dbl)
                        n4434 = local read "avpp"() -> (w1288:i32)
                        n4435 = call "tt_timeandsamples.vi"("bin"=w1282, "refreshtime"=w1276, "srateAODOtt"=w1279, "tot#ofsamples"=w1284) -> ("refreshrate"=w1280:dbl, "refreshbuffer"=w1281:i32, "timetracecycles"=w1286:i32)  [unwired: 5 in]
                        n4436 = local read "bin"() -> (w1283:dbl)
                        n4437 = call "2pparameters.vi"("command"="get") -> ("params out"=w1295:T12)  [unwired: 1 in]
                        n4438 = Bundle By Name(cluster=w1295, "Drawing Mode"=w1268, "measpoints"=w1284, "tt_cycles"=w1286, "refreshbuffer"=w1281, "refreshrate"=w1280, "Vx-ref"=w1287, "Vy-ref"=w1289, "srate"=w1278, "finite"=w1291, "cont"=w1290, "wavdet"=w1292, "avpp"=w1288, "srateAODO"=w1285, "bufferAI"=w1281, "bin"=w1283, "Angle Img"=w1275, "Vxminref"=w1274, "Vxmaxref"=w1273, "Vyminref"=w1272, "Vymaxref"=w1271, "Xpixels Img"=w1270, "Ypixels Img"=w1269, "Pel"=w1267, "Vz-reset"=0.0, "AIoverride"=w1265, "type"="Lifetime (contour)") -> (w1293:T12)
                        n4439 = Reciprocal(x=w1280) -> (1/x=w1277:dbl)
                        n4440 = local write "refreshtime"(w1277) -> ()
                        n4441 = call "2pparameters.vi"("Params in"=w1293, "command"="set") -> ()  [unwired: 1 out]
                      }
                      frame "X-Y-Z-t movie" {
                      }
                      frame "linescan" {
                      }
                      frame "Timetrace" {
                        n4442 = local read "Vy-min draw"() -> (w1305:dbl)
                        n4443 = local read "Vy-max draw"() -> (w1304:dbl)
                        n4444 = local read "Vx-min draw"() -> (w1307:dbl)
                        n4445 = local read "Vx-max draw"() -> (w1306:dbl)
                        n4446 = local read "xpixels ref"() -> (w1303:i32)
                        n4447 = local read "ypixels ref"() -> (w1302:i32)
                        n4448 = local read "ROI Type"() -> (w1301:u16)
                        n4449 = local read "srateAODOtt"() -> (w1312:dbl)
                        n4450 = local read "# of frames"() -> (w1317:i32)
                        n4451 = local read "refreshtime"() -> (w1309:dbl)
                        n4452 = local read "Pel"() -> (w1300:dbl)
                        n4453 = local read "bin"() -> (w1315:dbl)
                        n4454 = local read "Override AI buffer"() -> (w1298:bool)
                        n4455 = local read "finite samples"() -> (w1324:bool)
                        n4456 = local read "srateAODOtt"() -> (w1311:dbl)
                        n4457 = local read "srateAODOtt"() -> (w1318:dbl)
                        n4458 = local read "continuous"() -> (w1323:bool)
                        n4459 = local read "Angle ref"() -> (w1308:dbl)
                        n4460 = local read "wavdet"() -> (w1325:bool)
                        n4461 = local read "Vx-ref"() -> (w1320:dbl)
                        n4462 = local read "Vy-ref"() -> (w1322:dbl)
                        n4463 = local read "avpp"() -> (w1321:i32)
                        n4464 = call "tt_timeandsamples.vi"("bin"=w1315, "refreshtime"=w1309, "srateAODOtt"=w1312, "tot#ofsamples"=w1317) -> ("refreshrate"=w1313:dbl, "refreshbuffer"=w1314:i32, "timetracecycles"=w1319:i32)  [unwired: 5 in]
                        n4465 = local read "bin"() -> (w1316:dbl)
                        n4466 = call "2pparameters.vi"("command"="get") -> ("params out"=w1328:T12)  [unwired: 1 in]
                        n4467 = Bundle By Name(cluster=w1328, "Drawing Mode"=w1301, "measpoints"=w1317, "tt_cycles"=w1319, "refreshbuffer"=w1314, "refreshrate"=w1313, "Vx-ref"=w1320, "Vy-ref"=w1322, "srate"=w1311, "finite"=w1324, "cont"=w1323, "wavdet"=w1325, "avpp"=w1321, "srateAODO"=w1318, "bufferAI"=w1314, "bin"=w1316, "Angle Img"=w1308, "Vxminref"=w1307, "Vxmaxref"=w1306, "Vyminref"=w1305, "Vymaxref"=w1304, "Xpixels Img"=w1303, "Ypixels Img"=w1302, "Pel"=w1300, "Vz-reset"=0.0, "AIoverride"=w1298, "type"="Timetrace") -> (w1326:T12)
                        n4468 = Reciprocal(x=w1313) -> (1/x=w1310:dbl)
                        n4469 = local write "refreshtime"(w1310) -> ()
                        n4470 = call "2pparameters.vi"("Params in"=w1326, "command"="set") -> ()  [unwired: 1 out]
                      }
                      frame "Lifetime (point)" {
                      }
                    }
                  }
                  frame #1 {
                    w1331 = FALSE ("wavdet")
                    n4471 = call "2pparameters.vi"("command"="get") -> ("params out"=w1335:T12)  [unwired: 1 in]
                    n4472 = Bundle By Name(cluster=w1335, "finite"=w1331, "cont"=w1331, "wavdet"=TRUE) -> (w1332:T12)
                    n4473 = call "2pparameters.vi"("Params in"=w1332, "command"="set") -> ()  [unwired: 1 out]
                  }
                  frame #2 {
                    n4474 = local read "Meastab"() -> (w1362:enum32{"X-Y Image", "Linescan", "Timetrace"})
                    n4475 = property on="AO channels" class="Ring (strict)"() -> ("RingText.Text"=w1337:string)  [unwired: 2 in, 2 out]
                    n4476 = property on="refwf" class="Ring (strict)"() -> ("RingText.Text"=w1361:string)  [unwired: 2 in, 2 out]
                    n4477 = local read "Build analog waveform tabs"() -> (w1360:enum32{"Square", "Triangle", "Matlab"})
                    n4478 = case shown="\"X-Y Image\", Default" w1362 {
                      tunnel: [w1368 w1369] -> w1359
                      frame "X-Y Image", Default {
                        n4479 = local read "Sampling rate"() -> (w1368:dbl)
                      }
                      frame "Timetrace" {
                        n4480 = local read "srateAODOtt"() -> (w1369:dbl)
                      }
                    }
                    n4481 = local read "Matlab waveform path"() -> (w1352:path)
                    n4482 = local read "Period (ms)"() -> (w1355:dbl)
                    n4483 = local read "Frequency"() -> (w1354:dbl)
                    n4484 = local read "Tri Repeats"() -> (w1353:dbl)
                    n4485 = local read "Repeats"() -> (w1358:dbl)
                    n4486 = local read "Cycles"() -> (w1357:dbl)
                    n4487 = local read "Pulses"() -> (w1356:dbl)
                    n4488 = call "matlabwfexistsdialogue.vi"("Matlab waveform path"=w1352) -> ("mtalab waveform path out"=w1351:path)
                    n4489 = call "wfsizecalc.vi"("Sampling frequency (Hz)"=w1359, "AOtab"=w1360, "reference waveforms to"=w1361, "channel"=w1337, "Repeats"=w1358, "Cycles"=w1357, "Matlab wave file"=w1351, "pulses"=w1356, "Period (ms)"=w1355, "Frequency"=w1354, "Tri Repeats"=w1353) -> ("total size GB"=w1346:dbl, "gigabytesize wf"=w1342:dbl)  [unwired: 3 in]
                    n4490 = Greater?(x=w1342, y=0.5) -> (0:w1343:bool)
                    n4491 = Number To Fractional String(number=w1342, width (-)=i16 3) -> (F-format string=w1348:string)  [unwired: 2 in]
                    n4492 = Number To Fractional String(number=w1346, width (-)=i16 4) -> (F-format string=w1347:string)  [unwired: 2 in]
                    n4493 = Concatenate Strings("this is a crude approximation:\nyou're about to create a  " ("message"), w1348, " GB waveform for a total of " ("string"), w1347, " GB. Are you sure?" ("string")) -> (w1344:string)
                    n4494 = case shown="True" w1343 {
                      tunnel: w1344 -> [_ w1367]
                      tunnel: [TRUE ("T button?") w1364] -> w1338
                      frame False {
                      }
                      frame True {
                        n4495 = Two Button Dialog(message=w1367, 1:"No, don't do this." ("Center Button Text (\"No\")"), 2:"Yes, continue. " ("Left Button Text (\"Yes\")")) -> (T button?=w1364:bool)
                      }
                    }
                  }
                  frame #3 {
                    n4496 = case shown="True" w1370 {
                      tunnel: [_ w1374] -> w1372
                      tunnel: [_ w1373] -> w1371
                      frame False {
                      }
                      frame True {
                        n4497 = local read "AO channels"() -> (w1376:u32)
                        n4498 = call "2pparameters.vi"("command"="get") -> ("params out"=w1378:T12)  [unwired: 1 in]
                        n4499 = Unbundle By Name(w1378) -> ("aAO"=w1377:u32[])
                        n4500 = Search 1D Array(1D array=w1377, element=w1376) -> (index of element=w1374:i32)  [unwired: 1 in]
                        n4501 = Greater?(x=w1374, y=-1) -> (0:w1373:bool)
                        n4502 = case shown="True" w1373 {
                          tunnel: w1374 -> [_ w1392]
                          frame False {
                          }
                          frame True {
                            n4503 = local read "Meastab"() -> (w1381:enum32{"X-Y Image", "Linescan", "Timetrace"})
                            n4504 = case shown="\"Timetrace\"" w1381 {
                              tunnel: [w1393 w1394] -> w1380
                              frame "X-Y Image", Default {
                                n4505 = local read "Sampling rate"() -> (w1393:dbl)
                              }
                              frame "Timetrace" {
                                n4506 = local read "srateAODOtt"() -> (w1394:dbl)
                              }
                            }
                            n4507 = local read "Start amplitude (V)"() -> (w1389:dbl)
                            n4508 = local read "phase shift (ms)"() -> (w1384:dbl)
                            n4509 = local read "Step size (V)"() -> (w1387:dbl)
                            n4510 = local read "Baseline (V)"() -> (w1388:dbl)
                            n4511 = local read "Period (ms)"() -> (w1385:dbl)
                            n4512 = local read "padding value"() -> (w1382:dbl)
                            n4513 = local read "Repeats"() -> (w1391:dbl)
                            n4514 = local read "Cycles"() -> (w1390:dbl)
                            n4515 = local read "DC (%)"() -> (w1386:dbl)
                            n4516 = local read "Pulses"() -> (w1383:dbl)
                            n4517 = call "replace AO square wf param.vi"("Baseline (V)"=w1388, "Start amplitude (V)"=w1389, "Cycles"=w1390, "Repeats"=w1391, "index of AO wave"=w1392, "Step size (V)"=w1387, "DC (%)"=w1386, "Sampling frequency (Hz)"=w1380, "Period (ms)"=w1385, "Cycle length (s)"=w1384, "Pulses"=w1383, "padding value"=w1382) -> ()  [unwired: 4 in]
                          }
                        }
                      }
                    }
                  }
                  frame #4 {
                    n4518 = case shown="True" w1395 {
                      tunnel: w1397 -> [_ w1399]
                      tunnel: w1396 -> [_ w1398]
                      frame False {
                      }
                      frame True {
                        n4519 = case shown="True" w1398 {
                          tunnel: w1399 -> [_ w1407]
                          frame False {
                          }
                          frame True {
                            n4520 = call "waveformparamsv2.vi"("command"="get") -> ("Params out"=w1421:T17)  [unwired: 4 in, 2 out]
                            n4521 = Unbundle By Name(w1421) -> ("AO parameters"=w1420:T18)
                            n4522 = local read "Meastab"() -> (w1402:enum32{"X-Y Image", "Linescan", "Timetrace"})
                            n4523 = case shown="\"Timetrace\"" w1402 {
                              tunnel: [w1423 w1424] -> w1411
                              frame "X-Y Image", Default {
                                n4524 = local read "Sampling rate"() -> (w1423:dbl)
                              }
                              frame "Timetrace" {
                                n4525 = local read "srateAODOtt"() -> (w1424:dbl)
                              }
                            }
                            n4526 = Index Array(array=w1420, index=w1407) -> (element=w1409:T19)
                            n4527 = call "waveformsAObuffer.vi"("command"="get") -> ("AO wf out"=w1408:waveform(dbl)[])  [unwired: 1 in]
                            n4528 = call "generateRampedSquareWave_fromAOparameters.vi"("AO params"=w1409) -> ("Waveform"=w1406:waveform(dbl))  [unwired: 1 out]
                            n4529 = property on="refwf" class="Ring (strict)"() -> ("RingText.Text"=w1410:string)  [unwired: 2 in, 2 out]
                            n4530 = Replace Array Subset(array=w1408, new element=w1406, index=w1407) -> (w1405:waveform(dbl)[])
                            n4531 = call "waveformsDObuffer.vi"("command"="get") -> ("DO wf out"=w1416:digitalwaveform[])  [unwired: 1 in]
                            n4532 = call "correctwaveformsizetemp.vi"("new sampling frequency (Hz)"=w1411, "start"=FALSE, "reference waveforms to"=w1410, "Analog waveforms in"=w1405, "stop"=FALSE, "Digital waveforms in"=w1416) -> ("analog wf out"=w1414:waveform(dbl)[], "Digital wf out"=w1412:digitalwaveform[], "measpoints"=w1403:i32)
                            n4533 = local read "wavdet"() -> (w1404:bool)
                            n4534 = local write "Analog Lines Plot"(w1414) -> ()
                            n4535 = call "GetNumCamFramesv2.vi"("Digital Waveform Graph"=w1412) -> ("Numeric"=w1413:i32)  [unwired: 10 in]
                            n4536 = local write "Digital Lines Plot"(w1412) -> ()
                            n4537 = call "waveformsAObuffer.vi"("AO wf in"=w1414, "command"="set") -> ()  [unwired: 1 out]
                            n4538 = call "waveformsDObuffer.vi"("DO wf in"=w1412, "command"="set") -> ()  [unwired: 1 out]
                            n4539 = local write "Total Camera Frames"(w1413) -> ()
                            n4540 = case shown="True" w1404 {
                              tunnel: w1403 -> [_ w1425]
                              frame False {
                              }
                              frame True {
                                n4541 = local write "# of frames"(w1425) -> ()
                              }
                            }
                          }
                        }
                      }
                    }
                  }
                  frame #5 {
                    w1427 = FALSE ("addAO")
                    n4542 = local read "finite samples"() -> (w1428:bool)
                    n4543 = local read "continuous"() -> (w1429:bool)
                    n4544 = local read "wavdet"() -> (w1430:bool)
                    n4545 = local write "changeAOsq"(w1427) -> ()
                    n4546 = case shown="True" w1426 {
                      frame False {
                      }
                      frame True {
                        n4547 = local write "not loaded"(FALSE ("not loaded")) -> ()
                      }
                    }
                    n4548 = property on="load changed AOsq" class="Bool (strict)"("Val(Sgnl)"=w1427) -> ()  [unwired: 2 in, 2 out]
                    n4549 = call "2pparameters.vi"("command"="get") -> ("params out"=w1433:T12)  [unwired: 1 in]
                    n4550 = Bundle By Name(cluster=w1433, "finite"=w1428, "cont"=w1429, "wavdet"=w1430) -> (w1431:T12)
                    n4551 = call "2pparameters.vi"("Params in"=w1431, "command"="set") -> ()  [unwired: 1 out]
                  }
                }
              }
            }
          }
          event "load changed AOtri": Value Change {
            n4552 = event-data() -> ("NewVal"=w1436:bool)  [unwired: 1 in, 5 out]
            n4553 = case shown="True" w1436 {
              frame False {
              }
              frame True {
                n4554 = stacked-sequence {
                  seq-local: [_ _ _ w1578 _ _] -> [_ _ _ _ w1599 _]
                  seq-local: [_ _ _ w1577 _ _] -> [_ _ _ _ w1598 _]
                  seq-local: [_ _ w1544 _ _ _] -> [_ _ _ w1576 w1597 w1628]
                  frame #0 {
                    n4555 = local read "Measurement"() -> (w1438:T4)
                    n4556 = local write "changeAOtri"(TRUE ("addAO")) -> ()
                    n4557 = case shown="\"X-Y-t movie\", Default" w1438 {
                      frame "X-Y-t movie", Default {
                        n4558 = local read "avpp"() -> (w1459:i32)
                        n4559 = local read "Angle ref"() -> (w1458:dbl)
                        n4560 = local read "ROI Type"() -> (w1457:u16)
                        n4561 = local read "xpixels ref"() -> (w1454:i32)
                        n4562 = local read "Vx-min ref"() -> (w1453:dbl)
                        n4563 = local read "Vx-max ref"() -> (w1452:dbl)
                        n4564 = local read "ypixels ref"() -> (w1450:i32)
                        n4565 = local read "Vy-min ref"() -> (w1451:dbl)
                        n4566 = local read "Vy-max ref"() -> (w1447:dbl)
                        n4567 = local read "Sampling rate"() -> (w1441:dbl)
                        n4568 = local read "finite samples"() -> (w1442:bool)
                        n4569 = local read "continuous"() -> (w1445:bool)
                        n4570 = local read "wavdet"() -> (w1446:bool)
                        n4571 = local read "# of frames"() -> (w1444:i32)
                        n4572 = local read "maxbufferAI"() -> (w1443:i32)
                        n4573 = local read "Override AI buffer"() -> (w1439:bool)
                        n4574 = call "2pparameters.vi"("command"="get") -> ("params out"=w1456:T12)  [unwired: 1 in]
                        n4575 = Bundle By Name(cluster=w1456, "type"="X-Y-t movie", "avpp"=w1459, "Angle Img"=w1458, "Xpixels Img"=w1454, "Vx-min Img"=w1453, "VX-max Img"=w1452, "Ypixels Img"=w1450, "Vy-min Img"=w1451, "Vy-max Img"=w1447, "srate"=w1441, "srate Img"=w1441, "finite"=w1442, "cont"=w1445, "wavdet"=w1446, "measpoints"=w1444, "maxbufferAI"=w1443, "Drawing Mode"=w1457, "Vz-reset"=0.0, "AIoverride"=w1439) -> (w1448:T12)
                        n4576 = call "2pparameters.vi"("Params in"=w1448, "command"="set") -> ()  [unwired: 1 out]
                      }
                      frame "X-Y-Z stack" {
                        n4577 = call "2pparameters.vi"("command"="get") -> ("params out"=w1463:T12)  [unwired: 1 in]
                        n4578 = Bundle By Name(cluster=w1463, "type"="X-Y-Z stack") -> (w1461:T12)
                        n4579 = call "2pparameters.vi"("Params in"=w1461, "command"="set") -> ()  [unwired: 1 out]
                      }
                      frame "Lifetime (scan)" {
                        n4580 = call "2pparameters.vi"("command"="get") -> ("params out"=w1468:T12)  [unwired: 1 in]
                        n4581 = Bundle By Name(cluster=w1468, "type"="Lifetime (scan)") -> (w1466:T12)
                        n4582 = call "2pparameters.vi"("Params in"=w1466, "command"="set") -> ()  [unwired: 1 out]
                      }
                      frame "Lifetime (contour)" {
                        n4583 = local read "Vy-min draw"() -> (w1478:dbl)
                        n4584 = local read "Vy-max draw"() -> (w1477:dbl)
                        n4585 = local read "Vx-min draw"() -> (w1480:dbl)
                        n4586 = local read "Vx-max draw"() -> (w1479:dbl)
                        n4587 = local read "xpixels ref"() -> (w1476:i32)
                        n4588 = local read "ypixels ref"() -> (w1475:i32)
                        n4589 = local read "ROI Type"() -> (w1474:u16)
                        n4590 = local read "srateAODOtt"() -> (w1485:dbl)
                        n4591 = local read "# of frames"() -> (w1490:i32)
                        n4592 = local read "refreshtime"() -> (w1482:dbl)
                        n4593 = local read "Pel"() -> (w1473:dbl)
                        n4594 = local read "bin"() -> (w1488:dbl)
                        n4595 = local read "Override AI buffer"() -> (w1471:bool)
                        n4596 = local read "finite samples"() -> (w1497:bool)
                        n4597 = local read "srateAODOtt"() -> (w1484:dbl)
                        n4598 = local read "srateAODOtt"() -> (w1491:dbl)
                        n4599 = local read "continuous"() -> (w1496:bool)
                        n4600 = local read "Angle ref"() -> (w1481:dbl)
                        n4601 = local read "wavdet"() -> (w1498:bool)
                        n4602 = local read "Vx-ref"() -> (w1493:dbl)
                        n4603 = local read "Vy-ref"() -> (w1495:dbl)
                        n4604 = local read "avpp"() -> (w1494:i32)
                        n4605 = call "tt_timeandsamples.vi"("bin"=w1488, "refreshtime"=w1482, "srateAODOtt"=w1485, "tot#ofsamples"=w1490) -> ("refreshrate"=w1486:dbl, "refreshbuffer"=w1487:i32, "timetracecycles"=w1492:i32)  [unwired: 5 in]
                        n4606 = local read "bin"() -> (w1489:dbl)
                        n4607 = call "2pparameters.vi"("command"="get") -> ("params out"=w1501:T12)  [unwired: 1 in]
                        n4608 = Bundle By Name(cluster=w1501, "Drawing Mode"=w1474, "measpoints"=w1490, "tt_cycles"=w1492, "refreshbuffer"=w1487, "refreshrate"=w1486, "Vx-ref"=w1493, "Vy-ref"=w1495, "srate"=w1484, "finite"=w1497, "cont"=w1496, "wavdet"=w1498, "avpp"=w1494, "srateAODO"=w1491, "bufferAI"=w1487, "bin"=w1489, "Angle Img"=w1481, "Vxminref"=w1480, "Vxmaxref"=w1479, "Vyminref"=w1478, "Vymaxref"=w1477, "Xpixels Img"=w1476, "Ypixels Img"=w1475, "Pel"=w1473, "Vz-reset"=0.0, "AIoverride"=w1471, "type"="Lifetime (contour)") -> (w1499:T12)
                        n4609 = Reciprocal(x=w1486) -> (1/x=w1483:dbl)
                        n4610 = local write "refreshtime"(w1483) -> ()
                        n4611 = call "2pparameters.vi"("Params in"=w1499, "command"="set") -> ()  [unwired: 1 out]
                      }
                      frame "X-Y-Z-t movie" {
                      }
                      frame "linescan" {
                      }
                      frame "Timetrace" {
                        n4612 = local read "Vy-min draw"() -> (w1511:dbl)
                        n4613 = local read "Vy-max draw"() -> (w1510:dbl)
                        n4614 = local read "Vx-min draw"() -> (w1513:dbl)
                        n4615 = local read "Vx-max draw"() -> (w1512:dbl)
                        n4616 = local read "xpixels ref"() -> (w1509:i32)
                        n4617 = local read "ypixels ref"() -> (w1508:i32)
                        n4618 = local read "ROI Type"() -> (w1507:u16)
                        n4619 = local read "srateAODOtt"() -> (w1518:dbl)
                        n4620 = local read "# of frames"() -> (w1523:i32)
                        n4621 = local read "refreshtime"() -> (w1515:dbl)
                        n4622 = local read "Pel"() -> (w1506:dbl)
                        n4623 = local read "bin"() -> (w1521:dbl)
                        n4624 = local read "Override AI buffer"() -> (w1504:bool)
                        n4625 = local read "finite samples"() -> (w1530:bool)
                        n4626 = local read "srateAODOtt"() -> (w1517:dbl)
                        n4627 = local read "srateAODOtt"() -> (w1524:dbl)
                        n4628 = local read "continuous"() -> (w1529:bool)
                        n4629 = local read "Angle ref"() -> (w1514:dbl)
                        n4630 = local read "wavdet"() -> (w1531:bool)
                        n4631 = local read "Vx-ref"() -> (w1526:dbl)
                        n4632 = local read "Vy-ref"() -> (w1528:dbl)
                        n4633 = local read "avpp"() -> (w1527:i32)
                        n4634 = call "tt_timeandsamples.vi"("bin"=w1521, "refreshtime"=w1515, "srateAODOtt"=w1518, "tot#ofsamples"=w1523) -> ("refreshrate"=w1519:dbl, "refreshbuffer"=w1520:i32, "timetracecycles"=w1525:i32)  [unwired: 5 in]
                        n4635 = local read "bin"() -> (w1522:dbl)
                        n4636 = call "2pparameters.vi"("command"="get") -> ("params out"=w1534:T12)  [unwired: 1 in]
                        n4637 = Bundle By Name(cluster=w1534, "Drawing Mode"=w1507, "measpoints"=w1523, "tt_cycles"=w1525, "refreshbuffer"=w1520, "refreshrate"=w1519, "Vx-ref"=w1526, "Vy-ref"=w1528, "srate"=w1517, "finite"=w1530, "cont"=w1529, "wavdet"=w1531, "avpp"=w1527, "srateAODO"=w1524, "bufferAI"=w1520, "bin"=w1522, "Angle Img"=w1514, "Vxminref"=w1513, "Vxmaxref"=w1512, "Vyminref"=w1511, "Vymaxref"=w1510, "Xpixels Img"=w1509, "Ypixels Img"=w1508, "Pel"=w1506, "Vz-reset"=0.0, "AIoverride"=w1504, "type"="Timetrace") -> (w1532:T12)
                        n4638 = Reciprocal(x=w1519) -> (1/x=w1516:dbl)
                        n4639 = local write "refreshtime"(w1516) -> ()
                        n4640 = call "2pparameters.vi"("Params in"=w1532, "command"="set") -> ()  [unwired: 1 out]
                      }
                      frame "Lifetime (point)" {
                      }
                    }
                  }
                  frame #1 {
                    w1537 = FALSE ("wavdet")
                    n4641 = call "2pparameters.vi"("command"="get") -> ("params out"=w1541:T12)  [unwired: 1 in]
                    n4642 = Bundle By Name(cluster=w1541, "finite"=w1537, "cont"=w1537, "wavdet"=TRUE) -> (w1538:T12)
                    n4643 = call "2pparameters.vi"("Params in"=w1538, "command"="set") -> ()  [unwired: 1 out]
                  }
                  frame #2 {
                    n4644 = local read "Meastab"() -> (w1568:enum32{"X-Y Image", "Linescan", "Timetrace"})
                    n4645 = property on="AO channels" class="Ring (strict)"() -> ("RingText.Text"=w1543:string)  [unwired: 2 in, 2 out]
                    n4646 = property on="refwf" class="Ring (strict)"() -> ("RingText.Text"=w1567:string)  [unwired: 2 in, 2 out]
                    n4647 = local read "Build analog waveform tabs"() -> (w1566:enum32{"Square", "Triangle", "Matlab"})
                    n4648 = case shown="\"X-Y Image\", Default" w1568 {
                      tunnel: [w1574 w1575] -> w1565
                      frame "X-Y Image", Default {
                        n4649 = local read "Sampling rate"() -> (w1574:dbl)
                      }
                      frame "Timetrace" {
                        n4650 = local read "srateAODOtt"() -> (w1575:dbl)
                      }
                    }
                    n4651 = local read "Matlab waveform path"() -> (w1558:path)
                    n4652 = local read "Period (ms)"() -> (w1561:dbl)
                    n4653 = local read "Frequency"() -> (w1560:dbl)
                    n4654 = local read "Tri Repeats"() -> (w1559:dbl)
                    n4655 = local read "Repeats"() -> (w1564:dbl)
                    n4656 = local read "Cycles"() -> (w1563:dbl)
                    n4657 = local read "Pulses"() -> (w1562:dbl)
